vi "Replace inputs and outputs.vi"() -> ()   [LabVIEW 2020]
uses:
  <vilib>/Utility/traverseref.llb/TRef TravTarget.ctl
  <vilib>/Utility/config.llb/Read Key (String).vi
  <vilib>/Utility/config.llb/NI_LVConfig.lvlib
panel:
  out "section exists?":bool
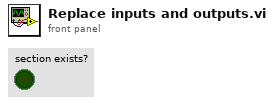
[diagram p1: front panel]
types:
  T1 = typedef "NI_LVConfig.lvlib/Config Data RefNum.ctl" = refnum<k1>
  T2 = typedef "TRef TravTarget.ctl" = enum16{"FP", "BD", "Other"}
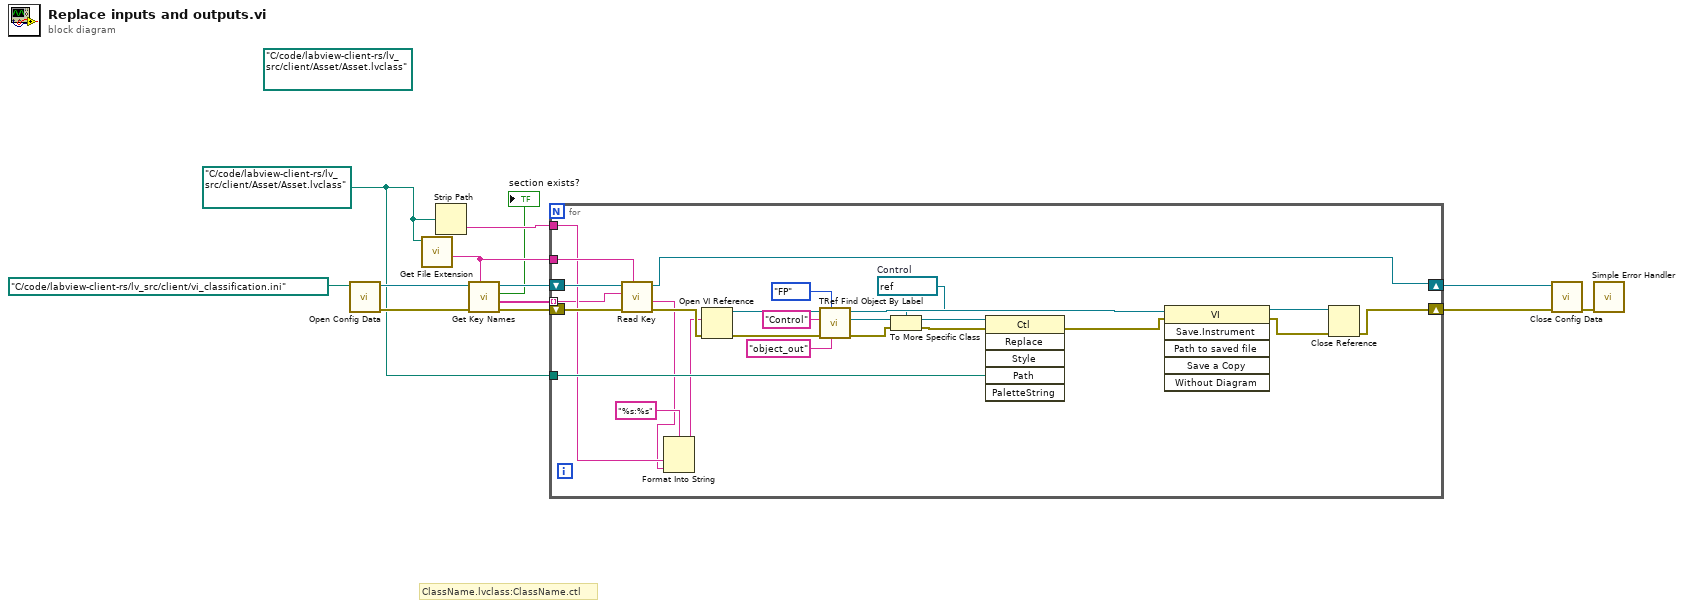
[diagram p0: block diagram]
diagram:
  (unwired) path "C:/code/labview-client-rs/lv_src/client/Asset/Asset.lvclass" ("Path")
  w1 = path "C:/code/labview-client-rs/lv_src/client/Asset/Asset.lvclass" ("Path")
  # "ClassName.lvclass:ClassName.ctl"
  n1 = call <vilib>:"Open Config Data.vi"("configuration file path"=path "C:/code/labview-client-rs/lv_src/client/vi_classification.ini") -> ("error out"=w11:errorcluster, "refnum"=w2:T1)  [unwired: 8 in, 1 out]
  n2 = call <vilib>:"Get File Extension.vi"("file"=w1) -> ("filename without extension"=w8:string)  [unwired: 6 in, 4 out]
  n3 = Strip Path(path=w1) -> (name=w6:string)  [unwired: 1 out]
  n4 = call <vilib>:"Get Key Names.vi"("section"=w8, "error in (no error)"=w11, "refnum"=w2) -> ("error out"=w7:errorcluster, "key names"=w10:string[], "section exists?"=→"section exists?":bool, "refnum out"=w9:T1)  [unwired: 5 in]
  n5 = for {
    tunnel: w10 -> [w17] mode=indexing
    tunnel: w8 -> [w25]
    tunnel: w6 -> [w18]
    shift-right: [w23] -> w5
    shift-left: w9 -> [w24]
    shift-right: [w21] -> w4
    shift-left: w7 -> [w22]
    tunnel: w1 -> [w26]
    w27 = refnum<vi> refnum  # Control
    n6 = call-poly <vilib>:"Read Key.vi"("section"=w25, "error in (no error)"=w22, "key"=w17, "refnum"=w24) -> ("error out"=w20:errorcluster, "value"=w15:string, "refnum out"=w23:T1)  [unwired: 4 in, 1 out]
    n7 = Format Into String(format string="%s:%s", w18, w15) -> (resulting string=w16:string)  [unwired: 2 in, 1 out]
    n8 = Open VI Reference(vi path=w16, error in (no error)=w20) -> (vi reference=w35:refnum<vi>, error out=w36:errorcluster)  [unwired: 4 in]
    n9 = call <vilib>:"TRef Find Object By Label.vi"("Label"="object_out", "Traverse Target"=TRef_TravTarget."FP", "error in (no error)"=w36, "Class Name"="Control", "VI Ref"=w35) -> ("error out"=w34:errorcluster, "Found Obj Ref"=w32:refnum<vi>, "dup VI Ref"=w37:refnum<vi>)  [unwired: 3 in, 1 out]
    n10 = To More Specific Class(target class=w27, reference=w32, error in=w34) -> (specific class reference=w33:refnum<vi>, error out=w39:errorcluster)
    n11 = invoke class="Ctl" method="Replace"(reference=w33, error in=w39, "Path"=w26) -> (error out=w38:errorcluster)  [unwired: 3 in, 5 out]
    n12 = invoke class="VI" method="Save.Instrument"(reference=w37, error in=w38) -> (reference out=w30:refnum<vi>, error out=w31:errorcluster)  [unwired: 4 in, 4 out]
    n13 = Close Reference(reference=w30, error in (no error)=w31) -> (error out=w21:errorcluster)
  }
  n14 = call <vilib>:"Close Config Data.vi"("error in (no error)"=w4, "refnum"=w5) -> ("error out"=w13:errorcluster)  [unwired: 8 in, 1 out]
  n15 = call <vilib>:"Simple Error Handler.vi"("error in (no error)"=w13) -> ()  [unwired: 4 in, 5 out]
